vi "LoadAllCtrlsConfig.vi"(7 "ExcludeLabels":string[](array[string])=[""], 11 "VI in":refnum<vi>) -> ()   [LabVIEW 2020]
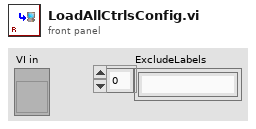
[diagram p1: front panel]
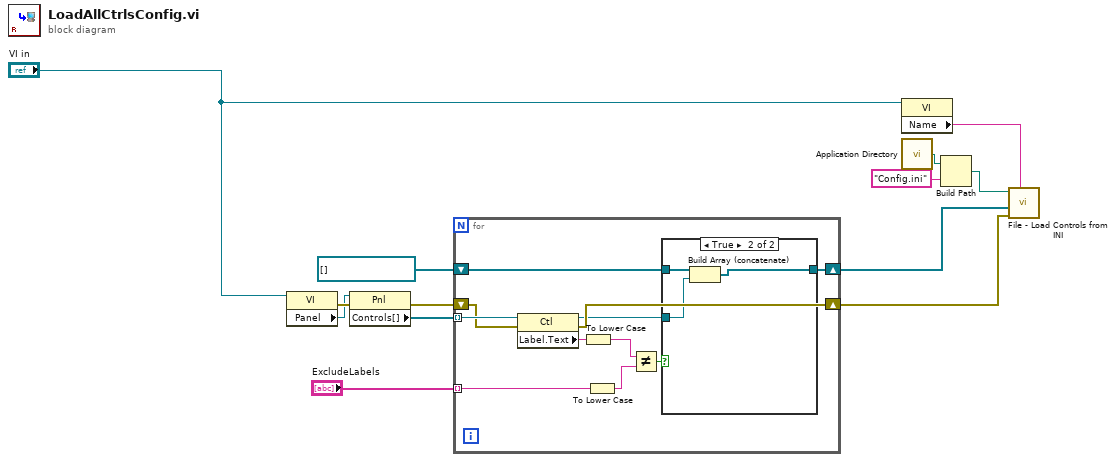
[diagram p0: block diagram]
diagram:
  n1 = property class="VI"(reference="VI in") -> (error out=w10:errorcluster, "Panel"=w9:refnum<vi>)  [unwired: 1 in, 1 out]
  n2 = property class="Pnl"(reference=w9, error in=w10) -> (error out=w6:errorcluster, "Controls[]"=w4:refnum<vi>[])  [unwired: 1 out]
  n3 = for {
    tunnel: w4 -> [w24] mode=indexing
    shift-right: [w21] -> w2
    shift-left: w6 -> [w22]
    tunnel: "ExcludeLabels" -> [w20] mode=indexing
    shift-right: [w14] -> w1
    shift-left: refnum<vi>[] [] ("Controls[]") -> [w15]
    n4 = property class="Ctl"(reference=w24, error in=w22) -> (reference out=w16:refnum<vi>, error out=w21:errorcluster, "Label.Text"=w23:string)
    n5 = To Lower Case(string=w23) -> (all lower case string=w19:string)
    n6 = To Lower Case(string=w20) -> (all lower case string=w18:string)
    n7 = Not Equal?(x=w19, y=w18) -> (x != y?=w17:bool)
    n8 = case shown="True" w17 {
      tunnel: w16 -> [_ w26]
      tunnel: w15 -> [w25 w28]
      tunnel: [w25 w27] -> w14
      frame False {
      }
      frame True {
        n9 = Build Array (concatenate)(w28, w26) -> (w27:refnum<vi>[])
      }
    }
  }
  n10 = property class="VI"(reference="VI in") -> ("Name"=w13:string)  [unwired: 1 in, 2 out]
  n11 = call <vilib>:"Application Directory.vi"() -> ("Application Directory"=w11:path)
  n12 = Build Path(base path=w11, name or relative path="Config.ini") -> (appended path=w8:path)
  n13 = call "File - Load Controls from INI.vi"("Section"=w13, "error in (no error)"=w2, "Array of References"=w1, "INI File"=w8) -> ()  [unwired: 7 in, 1 out]
